vi "kousei.vi"(6 "timeout (ms)(10000)":i32=10000, 7 "Application ID":string, 8 "error in (no error)":errorcluster caption="エラー入力 (エラーなし)", 11 "Input Text":string) -> (0 "Error out":errorcluster caption="エラー出力", 3 "Suggestion":T1[](array[typedef]))   [LabVIEW 2015, in "LV-Proof-Reading.lvlib"]
doc: "Web Services by Yahoo! JAPAN ( https://developer.yahoo.co.jp/sitemap/)"
uses:
  LV-Proof-Reading.lvlib
  suggestion.ctl
  <vilib>/httpClient/POSTBuffer.vi
  <vilib>/httpClient/LabVIEWHTTPClient.lvlib
panel:
  out "POST Data":string
  out "headers":string
  out "body":string
  # "Yahoo 校正支援 API"
  # "Response"
  # "Web Services by Yahoo! JAPAN ( https://developer.yahoo.co.jp/sitemap/)"
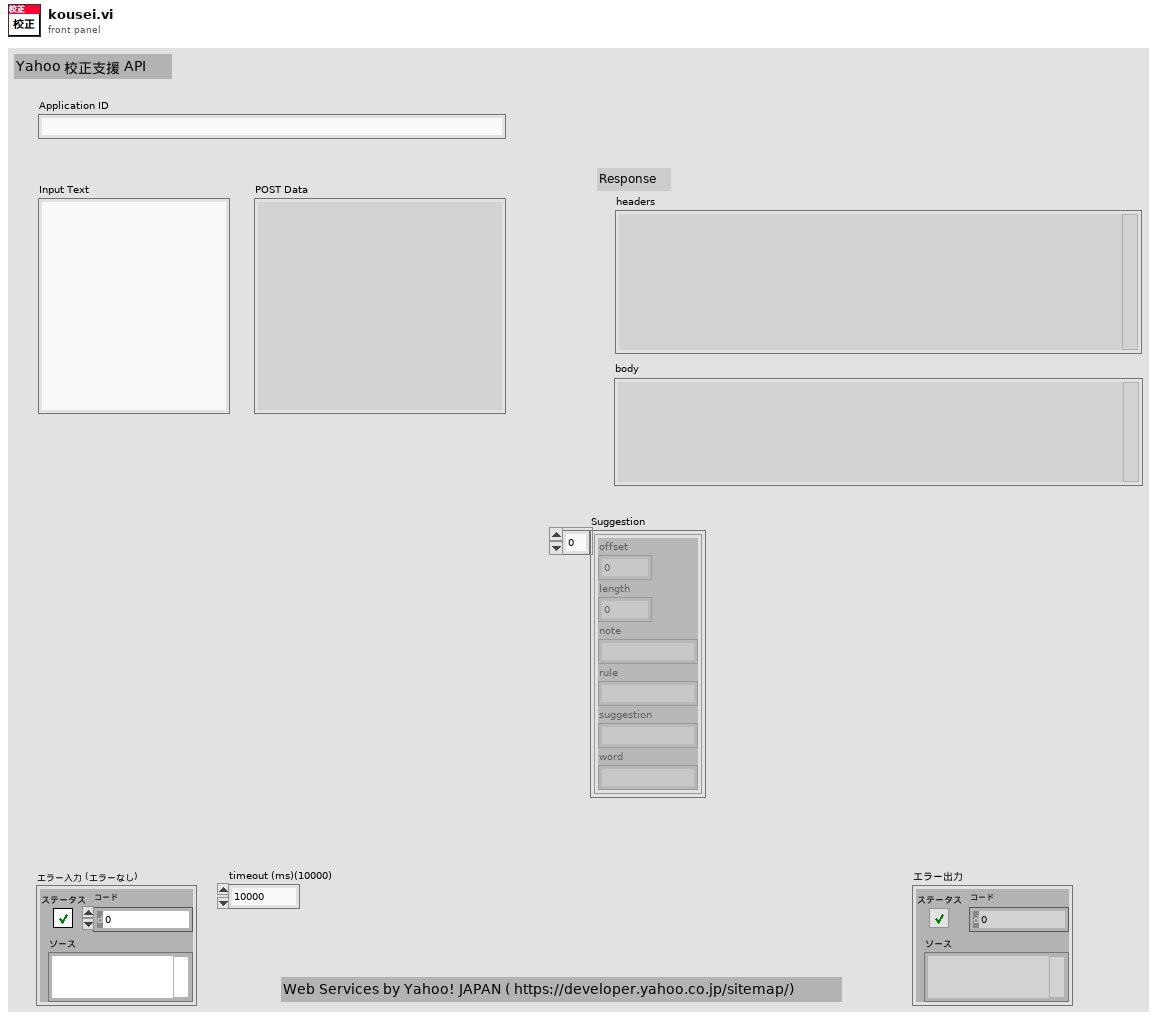
[diagram p1: front panel]
types:
  T1 = typedef "LV-Proof-Reading.lvlib/suggestion.ctl" = cluster{"offset":i32, "length":i32, "note":string, "rule":string, "suggestion":string, "word":string}
  T2 = typedef "LabVIEWHTTPClient.lvlib/ClientHandle.ctl" = refnum<k1>
  T3 = typedef "LV-Proof-Reading.lvlib/kousei - Response Data JSON.ctl" = cluster{"id":string, "jsonrpc":string, "result":cluster{"suggestions":cluster{"length":string, "note":string, "offset":string, "rule":string, "suggestion":string, "word":string}[]}}
  T4 = cluster{"length":string, "note":string, "offset":string, "rule":string, "suggestion":string, "word":string}[]
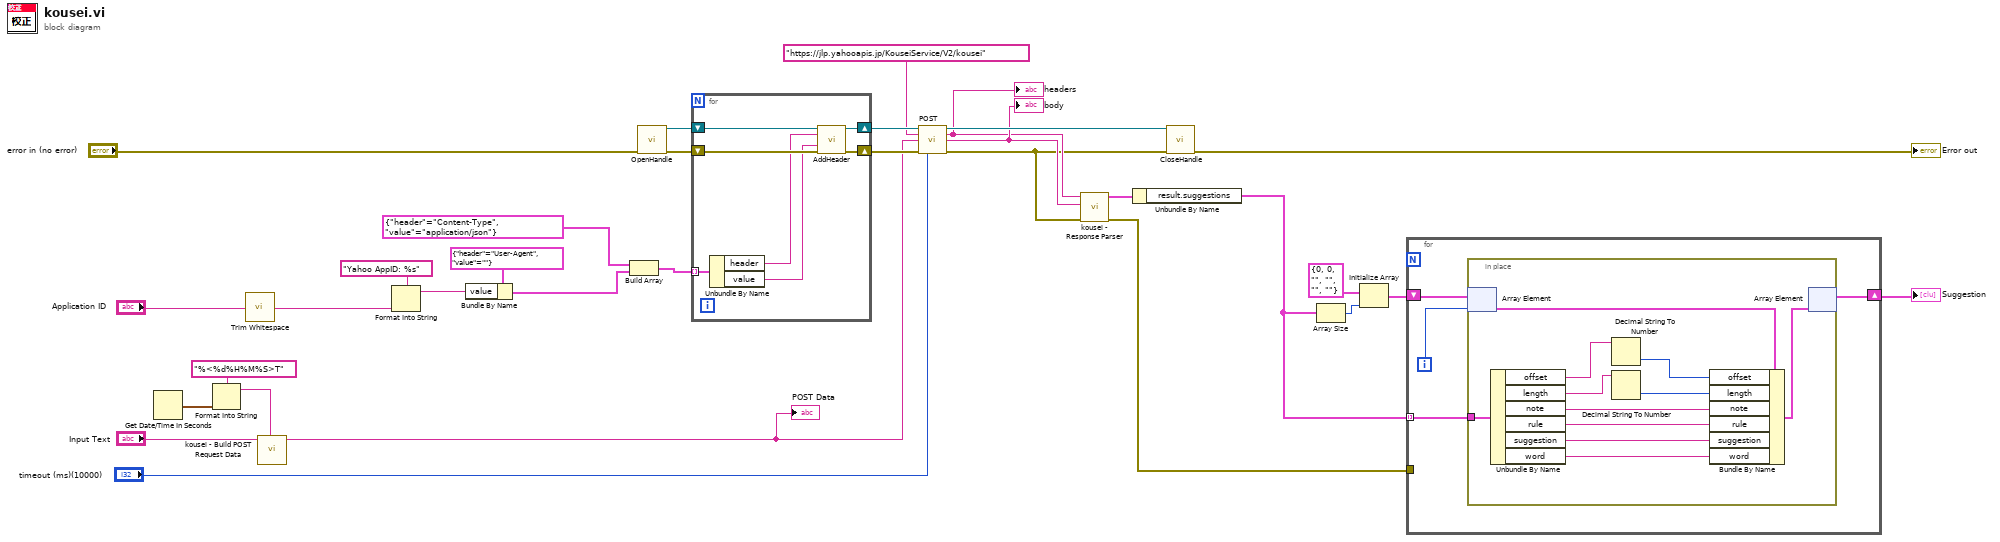
[diagram p0: block diagram]
diagram:
  n1 = Get Date/Time In Seconds() -> (seconds since 1Jan1904=w15:timestamp)
  n2 = Format Into String(format string="%<%d%H%M%S>T", w15) -> (resulting string=w13:string)  [unwired: 2 in, 1 out]
  n3 = call <vilib>:"Trim Whitespace.vi"("string"="Application ID") -> ("trimmed string"=w1:string)  [unwired: 1 in]
  n4 = call "kousei - Build POST Request Data.vi"("Request ID"=w13, "Input Text"="Input Text") -> ("JSON string"=w22:string)  [unwired: 8 in, 1 out]
  "POST Data" <- w22
  n5 = Format Into String(format string="Yahoo AppID: %s", w1) -> (resulting string=w17:string)  [unwired: 2 in, 1 out]
  n6 = Bundle By Name(cluster=cluster{"header":string, "value":string} {"header"="User-Agent", "value"=""} ("Cluster"), "value"=w17) -> (w16:cluster{"header":string, "value":string})
  n7 = Build Array(cluster{"header":string, "value":string} {"header"="Content-Type", "value"="application/json"} ("Cluster"), w16) -> (w27:cluster{"header":string, "value":string}[])
  n8 = call <vilib>:"OpenHandle.vi"("error in (no error)"="error in (no error)") -> ("client handle out"=w32:T2, "error out"=w31:errorcluster)  [unwired: 13 in]
  n9 = for {
    shift-right: [w37] -> w30
    shift-left: w32 -> [w39]
    shift-right: [w36] -> w29
    shift-left: w31 -> [w38]
    tunnel: w27 -> [w35] mode=indexing
    n10 = Unbundle By Name(w35) -> ("header"=w34:string, "value"=w33:string)
    n11 = call <vilib>:"AddHeader.vi"("client handle"=w39, "header"=w34, "value"=w33, "error in (no error)"=w38) -> ("client handle out"=w37:T2, "error out"=w36:errorcluster)  [unwired: 10 in]
  }
  n12 = call-poly <vilib>:"POST.vi"("client handle"=w30, "url"="https://jlp.yahooapis.jp/KouseiService/V2/kousei", "buffer"=w22, "error in (no error)"=w29, "timeout (10000)"="timeout (ms)(10000)") -> ("client handle out"=w28:T2, "headers"=w4:string, "body"=w11:string, "error out"=w2:errorcluster)  [unwired: 7 in]
  "body" <- w11
  "headers" <- w4
  n13 = call "kousei - Response Parser.vi"("error in (no error)"=w2, "body"=w11, "headers"=w4) -> ("error out"=w3:errorcluster, "Response"=w10:T3)  [unwired: 7 in]
  n14 = Unbundle By Name(w10) -> ("result.suggestions"=w8:T4)
  n15 = call <vilib>:"CloseHandle.vi"("client handle"=w28, "error in (no error)"=w2) -> ("error out"=→"Error out":errorcluster)  [unwired: 13 in]
  n16 = Array Size(array=w8) -> (size(s)=w7:i32)
  n17 = Initialize Array(T1 {"offset"=0, "length"=0, "note"="", "rule"="", "suggestion"="", "word"=""} ("suggestions"), w7) -> (w6:T1[])
  n18 = for {
    tunnel: w8 -> [w40] mode=indexing
    shift-right: [w41] -> w5
    shift-left: w6 -> [w43]
    tunnel: w3 -> [_]
    i -> [w42]
    n19 = in-place {
      in-place-border: w40 -> [w52]
      n20 = in-place-array #1(w43, w42) -> (w54:T1)
      n21 = Unbundle By Name(w52) -> ("offset"=w47:string, "length"=w45:string, "note"=w48:string, "rule"=w49:string, "suggestion"=w50:string, "word"=w51:string)
      n22 = Decimal String To Number(string=w47) -> (number=w46:i32)  [unwired: 2 in, 1 out]
      n23 = Decimal String To Number(string=w45) -> (number=w44:i32)  [unwired: 2 in, 1 out]
      n24 = Bundle By Name(cluster=w54, "offset"=w46, "length"=w44, "note"=w48, "rule"=w49, "suggestion"=w50, "word"=w51) -> (w53:T1)
      n25 = in-place-array #1(w53) -> (w41:T1[])  [unwired: 1 out]
    }
  }
  "Suggestion" <- w5
